vi "Reset Assert Factory.vi"(8 "error in (no error)":errorcluster) -> (0 "error out":errorcluster)   [LabVIEW 2013, in "Caraya.lvlib" / "Assert Factory Manager.lvclass"]
doc: "Resets the Assert Factory implementation to the default value."
uses:
  Assert Factory Manager.lvclass
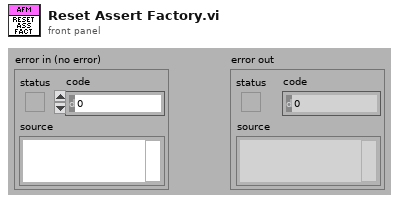
[diagram p1: front panel]
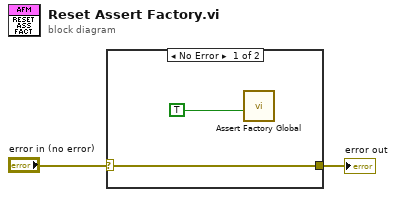
[diagram p0: block diagram]
diagram:
  n1 = case shown="No Error" "error in (no error)" {
    selector: "error in (no error)" -> [w4 w5]
    tunnel: [w4 w5] -> w1
    frame No Error {
      n2 = call "Assert Factory Global.vi"("Clear (F)"=TRUE ("Set (F)")) -> ()  [unwired: 8 in, 3 out]
    }
    frame Error {
    }
  }
  "error out" <- w1
